vi "Read Stored Values.vi"(8 "error in (no error)":errorcluster, 11 "APU Setup File in":T1) -> (0 "error out":errorcluster, 3 "Stored Values":dbl[](array[numeric]))   [LabVIEW 2018, in "RT - Analysis.lvlib"]
uses:
  RT - Analysis.lvlib
  Top Level/Shared Controls/APU Setup File.ctl
  Top Level/Shared VIs/Val Change Checker.vi
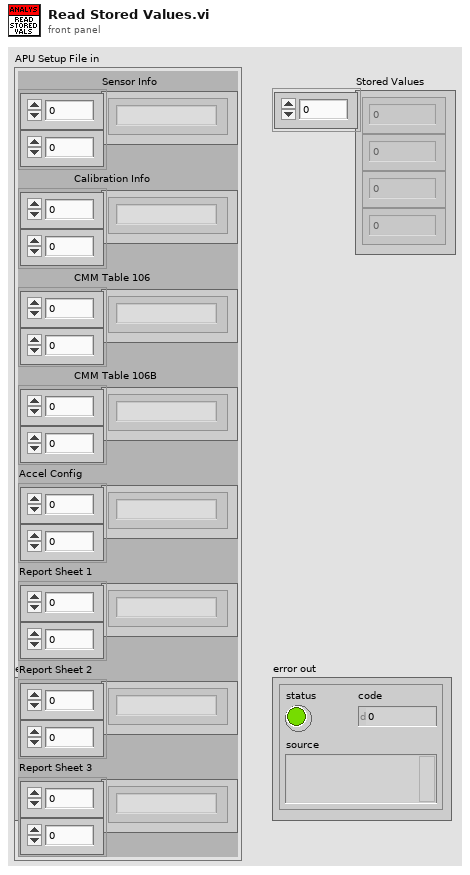
[diagram p1: front panel]
types:
  T1 = typedef "APU Setup File.ctl" = cluster{"Sensor Info":string[][], "Calibration Info":string[][], "CMM Table 106":string[][], "CMM Table 106B ":string[][], "Accel Config":string[][], "Report Sheet 1":string[][], "Report Sheet 2":string[][], "Report Sheet 3":string[][]}
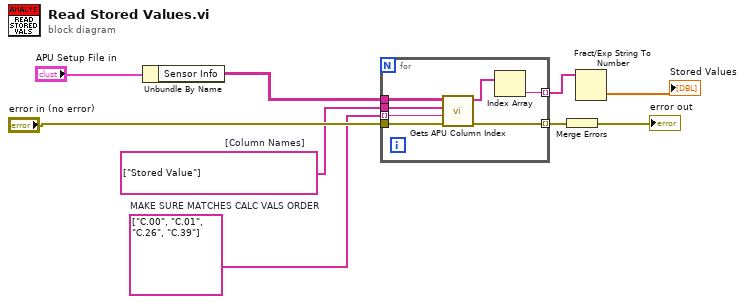
[diagram p0: block diagram]
diagram:
  w1 = string[] ["C.00", "C.01", "C.26", "C.39"]  # MAKE SURE MATCHES CALC VALS ORDER
  w3 = string[] ["Stored Value"]  # [Column Names]
  n1 = Unbundle By Name("APU Setup File in") -> ("Sensor Info"=w5:string[][])
  n2 = for {
    tunnel: w5 -> [w16]
    tunnel: w1 -> [w13] mode=indexing
    tunnel: "error in (no error)" -> [w14]
    tunnel: [w15] -> w4 mode=indexing
    tunnel: w3 -> [w12]
    tunnel: [w10] -> w2 mode=indexing
    n3 = call "Gets APU Column Index.vi"("error in (no error)"=w14, "Tag OR Name"=w13, "[Column Names]"=w12, "[[Array of Info]]"=w16) -> ("error out"=w15:errorcluster, "[Values out]"=w11:string[])  [unwired: 3 in, 3 out]
    n4 = Index Array(array=w11) -> (element=w10:string)  [unwired: 1 in]
  }
  n5 = Merge Errors(w4) -> (→"error out":errorcluster)
  n6 = Fract/Exp String To Number(string=w2) -> (number=→"Stored Values":dbl[])  [unwired: 3 in, 1 out]
